vi "GetPlots.vi"(2 "Sampled Signal":dbl[](array[numeric]), 3 "Two Level Signal":i16[][](array[numeric]), 4 "Sinusoidal Pattern":dbl[](array[numeric]), 5 "No. of Oversamples":i32) -> (0 "Sampled vs Continuous Signal":dbl[][](array[numeric]), 1 "Delta Sigma Modulation Signal":dbl[][](array[numeric]))   [LabVIEW 2014]
uses:
  <vilib>/gmath/NI_Gmath.lvlib
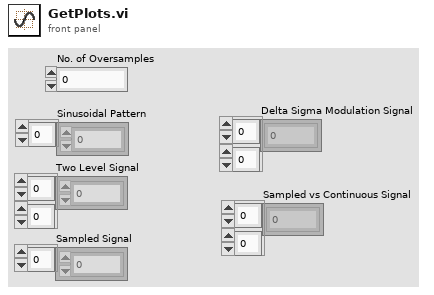
[diagram p1: front panel]
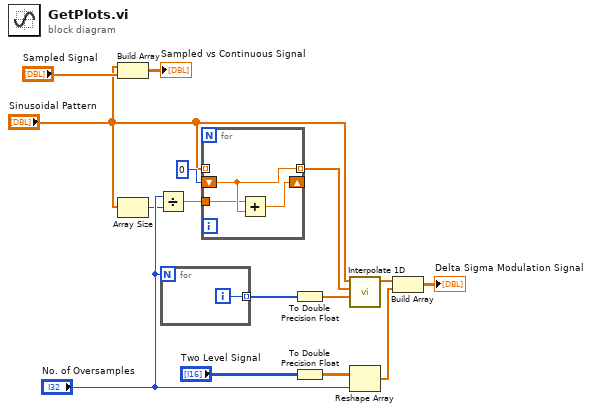
[diagram p0: block diagram]
diagram:
  n1 = Build Array("Sinusoidal Pattern", "Sampled Signal") -> (→"Sampled vs Continuous Signal":dbl[][])
  n2 = Array Size(array="Sinusoidal Pattern") -> (size(s)=w3:i32)
  n3 = Divide(x="No. of Oversamples", y=w3) -> (x/y=w2:dbl)
  n4 = for {
    N: "No. of Oversamples" -> [_]
    tunnel: [w16] -> w12 mode=indexing
    i -> [w16]
  }
  n5 = for {
    tunnel: "Sinusoidal Pattern" -> [_] mode=indexing
    shift-right: [w19] -> _
    shift-left: 0 -> [w18]
    tunnel: [w18] -> w1 mode=indexing
    tunnel: w2 -> [w17]
    n6 = Add(x=w17, y=w18) -> (x+y=w19:dbl)
  }
  n7 = To Double Precision Float(number=w12) -> (double precision float=w13:dbl[])
  n8 = To Double Precision Float(number="Two Level Signal") -> (double precision float=w10:dbl[][])
  n9 = call <vilib>:"Interpolate 1D.vi"("xi"=w13, "X"=w1, "Y"="Sinusoidal Pattern") -> ("yi"=w14:dbl[])  [unwired: 6 in, 2 out]
  n10 = Reshape Array(w10, "No. of Oversamples") -> (w11:dbl[])
  n11 = Build Array(w14, w11) -> (→"Delta Sigma Modulation Signal":dbl[][])
